vi "__FilterSet_Init.vi"(4 "EIDRef 2":refnum<vi>[](array[refnum]), 6 "IDRef 2":refnum<vi>[](array[refnum]), 7 "ParamIn":cluster{"mode":u8, "AccCode":u32, "AccMask":u32}, 8 "error in (no error)":errorcluster, 9 "EIDRef":refnum<vi>[](array[refnum]), 10 "IDRef":refnum<vi>[](array[refnum]), 11 "CtrlRef":T1) -> (0 "error out":errorcluster)   [LabVIEW 2011]
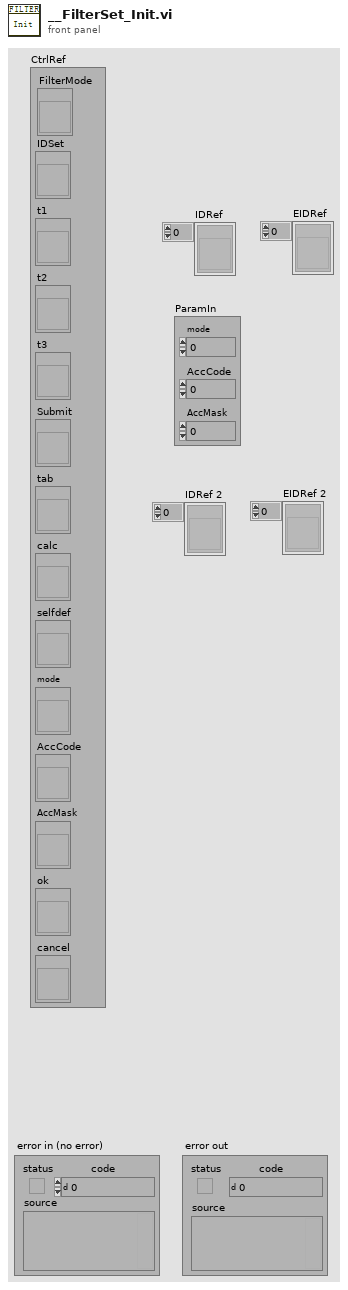
[diagram p1: front panel]
types:
  T1 = cluster{"FilterMode":refnum<vi>, "IDSet":refnum<vi>, "t1":refnum<vi>, "t2":refnum<vi>, "t3":refnum<vi>, "Submit":refnum<vi>, "tab":refnum<vi>, "calc":refnum<vi>, "selfdef":refnum<vi>, "mode":refnum<vi>, "AccCode":refnum<vi>, "AccMask":refnum<vi>, "ok":refnum<vi>, "cancel":refnum<vi>}
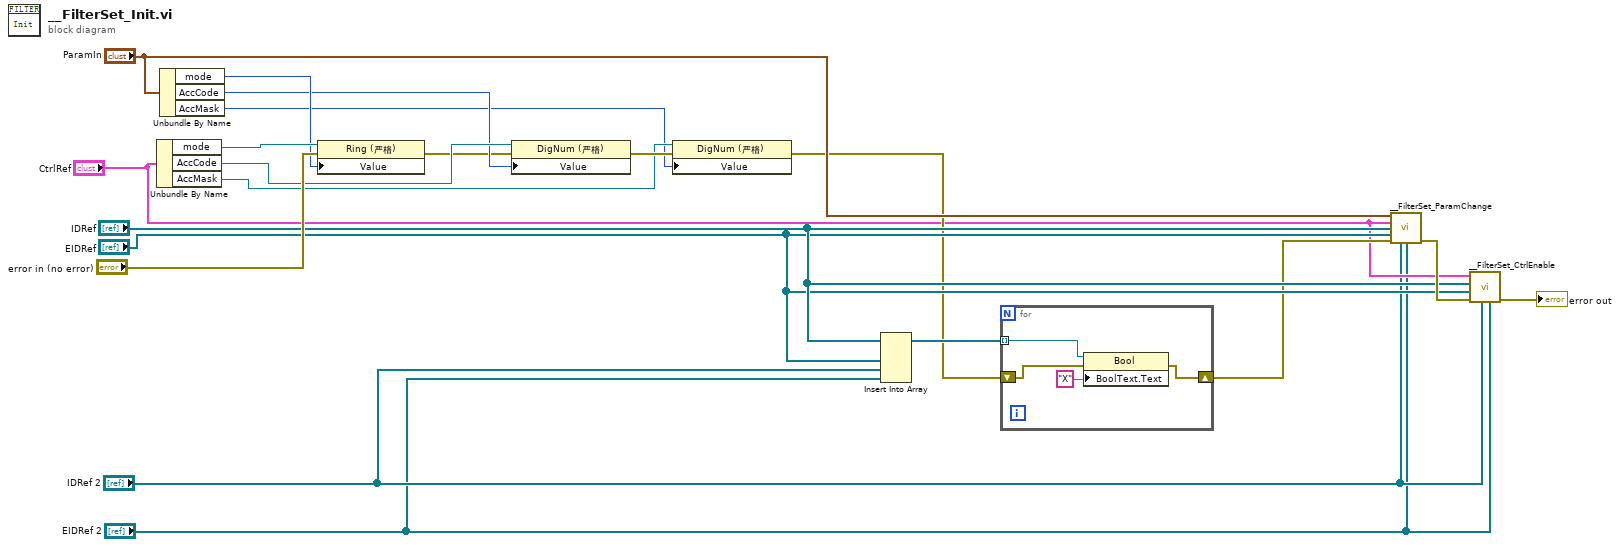
[diagram p0: block diagram]
diagram:
  n1 = Unbundle By Name("CtrlRef") -> ("mode"=w20:refnum<vi>, "AccCode"=w17:refnum<vi>, "AccMask"=w13:refnum<vi>)
  n2 = Unbundle By Name("ParamIn") -> ("mode"=w18:u8, "AccCode"=w16:u32, "AccMask"=w12:u32)
  n3 = property class="Ring (严格)"(reference=w20, error in="error in (no error)", "Value"=w18) -> (error out=w15:errorcluster)  [unwired: 1 out]
  n4 = property class="DigNum (严格)"(reference=w17, error in=w15, "Value"=w16) -> (error out=w14:errorcluster)  [unwired: 1 out]
  n5 = property class="DigNum (严格)"(reference=w13, error in=w14, "Value"=w12) -> (error out=w5:errorcluster)  [unwired: 1 out]
  n6 = Insert Into Array(array="IDRef", new element #1="EIDRef", new element #2="IDRef 2", new element #3="EIDRef 2") -> (w6:refnum<vi>[])  [unwired: 1 in]
  n7 = for {
    tunnel: w6 -> [w24] mode=indexing
    shift-right: [w22] -> w4
    shift-left: w5 -> [w23]
    n8 = property class="Bool"(reference=w24, error in=w23, "BoolText.Text"="X" ("布尔文本.文本")) -> (error out=w22:errorcluster)  [unwired: 1 out]
  }
  n9 = call "__FilterSet_ParamChange.vi"("Param in"="ParamIn", "CtrlRef"="CtrlRef", "IDRef"="IDRef", "EIDRef"="EIDRef", "error in (no error)"=w4, "IDRef 2"="IDRef 2", "EIDRef 2"="EIDRef 2") -> ("error out"=w10:errorcluster)  [unwired: 7 in, 1 out]
  n10 = call "__FilterSet_CtrlEnable.vi"("EIDRef 2"="EIDRef 2", "IDRef 2"="IDRef 2", "error in (no error)"=w10, "EIDRef"="EIDRef", "IDRef"="IDRef", "CtrlRef"="CtrlRef") -> ("error out"=→"error out":errorcluster)  [unwired: 5 in]
